vi "session_compression.vi"() -> ()   [LabVIEW 2013]
doc: "Illustrates how to enable compression for a session."
uses:
  libssh2/libssh2_flag.ctl
  libssh2/libssh2_method_type.ctl
  libssh2/libssh2_init_default.vi
  libssh2/libssh2_session_handshake_tcp.vi
  libssh2/libssh2.lvlib
panel:
  out "Compression Method (Server->Client)":string
  out "Compression Method (Client->Server)":string
  in  "hostname":string="localhost"
  out "error out":errorcluster
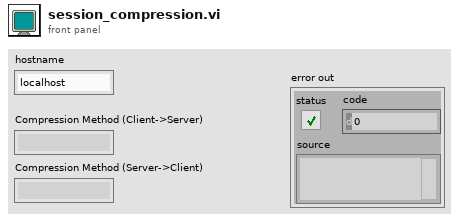
[diagram p1: front panel]
types:
  T1 = typedef "libssh2.lvlib/libssh2_method_type.ctl" = enum16{"LIBSSH2_METHOD_KEX", "LIBSSH2_METHOD_HOSTKEY", "LIBSSH2_METHOD_CRYPT_CS", "LIBSSH2_METHOD_CRYPT_SC", "LIBSSH2_METHOD_MAC_CS", "LIBSSH2_METHOD_MAC_SC", "LIBSSH2_METHOD_COMP_CS", "LIBSSH2_METHOD_COMP_SC", "LIBSSH2_METHOD_LANG_CS", "LIBSSH2_METHOD_LANG_SC", "LIBSSH2_METHOD_SIGN_ALGO"}
  T2 = typedef "libssh2.lvlib/libssh2_flag.ctl" = enum16{"SIGPIPE", "COMPRESS", "QUOTE_PATHS"}
  T3 = typedef "libssh2.lvlib/Session Refnum.ctl" = refnum<k1>
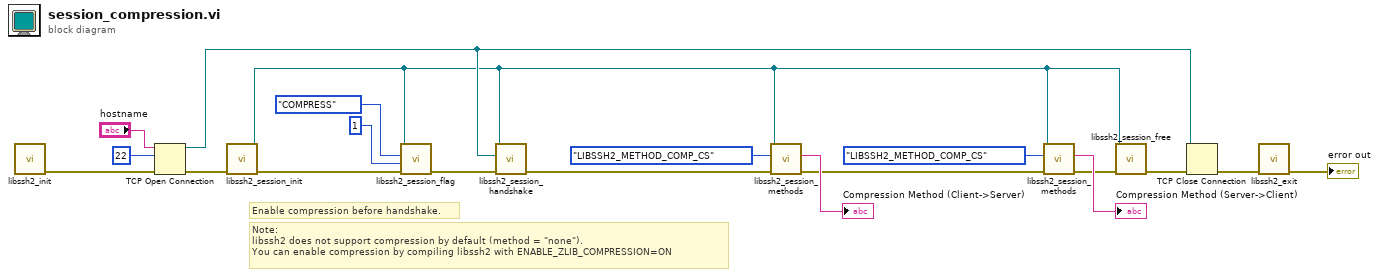
[diagram p0: block diagram]
diagram:
  # "Note:\nlibssh2 does not support compression by default (method = \"none\").\nYou can enable compression by compiling libssh2 with ENABLE_ZLIB_COMPRESSION=ON"
  # "Enable compression before handshake."
  n1 = call-poly "libssh2_init.vi"() -> ("error out"=w16:errorcluster)  [unwired: 11 in]
  n2 = TCP Open Connection(address="hostname", remote port or service name=u16 22, error in (no error)=w16) -> (connection ID=w10:refnum<k5>, error out=w15:errorcluster)  [unwired: 2 in]
  n3 = call "libssh2_session_init.vi"("error in (no error)"=w15) -> ("error out"=w18:errorcluster, "session"=w1:T3)  [unwired: 9 in]
  n4 = call "libssh2_session_flag.vi"("error in (no error)"=w18, "value (0 = disabled)"=1, "flag"=libssh2_flag."COMPRESS", "session"=w1) -> ("error out"=w13:errorcluster)  [unwired: 7 in]
  n5 = call-poly "libssh2_session_handshake.vi"("error in (no error)"=w13, "tcp connection"=w10, "session"=w1) -> ("error out"=w8:errorcluster)  [unwired: 8 in]
  n6 = call "libssh2_session_methods.vi"("error in (no error)"=w8, "method_type"=libssh2_method_type."LIBSSH2_METHOD_COMP_CS", "session"=w1) -> ("error out"=w3:errorcluster, "methods"=→"Compression Method (Client->Server)":string)  [unwired: 7 in]
  n7 = call "libssh2_session_methods.vi"("error in (no error)"=w3, "method_type"=libssh2_method_type."LIBSSH2_METHOD_COMP_CS", "session"=w1) -> ("error out"=w2:errorcluster, "methods"=→"Compression Method (Server->Client)":string)  [unwired: 7 in]
  n8 = call "libssh2_session_free.vi"("error in (no error)"=w2, "session"=w1) -> ("error out"=w12:errorcluster)  [unwired: 9 in]
  n9 = TCP Close Connection(connection ID=w10, error in (no error)=w12) -> (error out=w11:errorcluster)  [unwired: 1 in, 1 out]
  n10 = call "libssh2_exit.vi"("error in (no error)"=w11) -> ("error out"=→"error out":errorcluster)  [unwired: 10 in]
